vi "Connect to device (if only one).vi"(8 "error in":errorcluster) -> (0 "error out":errorcluster)   [LabVIEW 2015]
uses:
  Calibration and Function folders.ctl
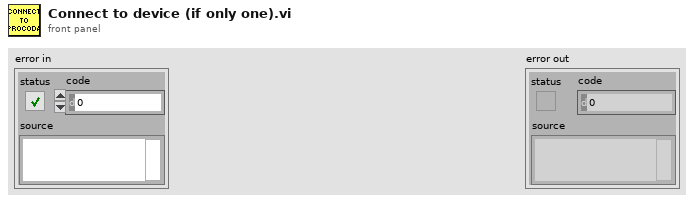
[diagram p1: front panel]
types:
  T1 = typedef "Calibration and Function folders.ctl" = enum16{"Sensors", "Functions", "Config File", "PublicAppFolder", "New ini File", "Set Config File", "Delete ini File"}
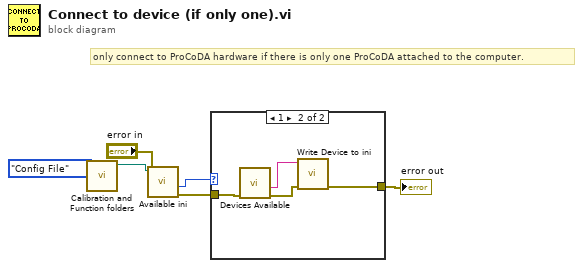
[diagram p0: block diagram]
diagram:
  # "only connect to ProCoDA hardware if there is only one ProCoDA attached to the computer."
  n1 = call "Calibration and Function folders.vi"("Folder"=Calibration_and_Function_folders."Config File") -> ("Selected Folder"=w6:path)  [unwired: 9 in, 1 out]
  n2 = call "Available ini.vi"("error in"="error in", "Config file path"=w6) -> ("error out"=w3:errorcluster, "Size"=w4:i32)  [unwired: 4 in, 4 out]
  n3 = case shown="1" w4 {
    tunnel: w3 -> [w7 w9]
    tunnel: [w7 w8] -> w2
    frame 0, Default {
    }
    frame 1 {
      n4 = call "Devices Available.vi"("error in (no error)"=w9) -> ("error out"=w10:errorcluster, "Default Device"=w11:tag)  [unwired: 6 in, 3 out]
      n5 = call "Write Device to ini.vi"("error in (no error)"=w10, "Device Name"=w11) -> ("error out"=w8:errorcluster)  [unwired: 9 in]
    }
  }
  "error out" <- w2
